vi "Info by Client ID.vi"(8 "error in (no error)":errorcluster, 10 "Node ID":u32, 11 "TCPMessageAPI in":refnum<class "TCPMessageAPI.lvclass">) -> (0 "error out":errorcluster, 2 "Client Info":T1, 3 "TCPMessageAPI out":refnum<class "TCPMessageAPI.lvclass">)   [LabVIEW 2020, in "Vecto.lvlib" / "TCPMessageAPI.lvclass"]
uses:
  TCPMessageAPI.lvclass
  Client Info.ctl
  proto/TcpClientHello/Data.ctl
  TCPMessageAPI.lvclass/TCPMessageAPI.ctl
  proto/TcpClientHello/TcpClientHello.lvlib
  Vecto.lvlib
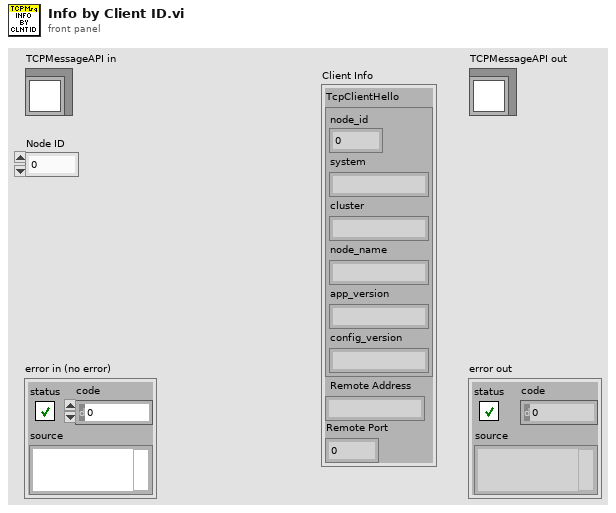
[diagram p1: front panel]
types:
  T1 = typedef "Vecto.lvlib/Client Info.ctl" = cluster{"TcpClientHello":T2, "Remote Address":string, "Remote Port":u16}
  T2 = typedef "TcpClientHello.lvlib/Data.ctl" = cluster{"node_id":u32, "system":string, "cluster":string, "node_name":string, "app_version":string, "config_version":string}
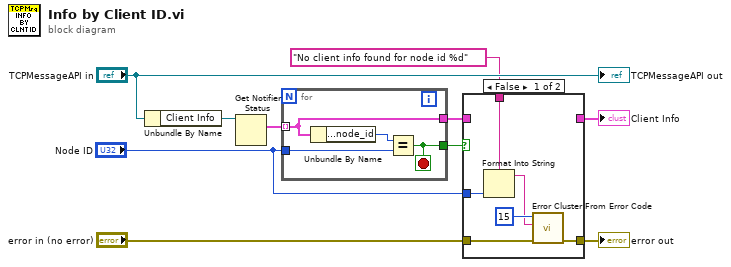
[diagram p0: block diagram]
diagram:
  n1 = Unbundle By Name("TCPMessageAPI in") -> ("Client Info"=w9:refnum<notifier>)
  n2 = Get Notifier Status(notifier=w9) -> (current notification=w1:T1[])  [unwired: 1 in, 4 out]
  n3 = for {
    tunnel: w1 -> [w11] mode=indexing
    tunnel: "Node ID" -> [w14]
    tunnel: [w11] -> w7
    tunnel: [w12] -> w8
    stop <- w12 stop-if-true
    n4 = Unbundle By Name(w11) -> ("TcpClientHello.node_id"=w13:u32)
    n5 = Equal?(x=w13, y=w14) -> (x = y?=w12:bool)
  }
  n6 = case shown="False" w8 {
    tunnel: w7 -> [_ w22]
    tunnel: [_ w22] -> w6
    tunnel: "error in (no error)" -> [w20 w21]
    tunnel: [w18 w21] -> w4
    tunnel: "Node ID" -> [w17 _]
    tunnel: "No client info found for node id %d" -> [w16 _]
    frame False {
      n7 = Format Into String(format string=w16, w17) -> (resulting string=w15:string)  [unwired: 2 in, 1 out]
      n8 = call <vilib>:"Error Cluster From Error Code.vi"("error in (no error)"=w20, "error message (\"\")"=w15, "error code (0)"=15) -> ("error out"=w18:errorcluster)  [unwired: 6 in]
    }
    frame True {
    }
  }
  "error out" <- w4
  "Client Info" <- w6
  "TCPMessageAPI out" <- "TCPMessageAPI in"
